vi "getIntersectionFromEnemy-BallLineAndGoalLine.vi"(8 "error in (no error)":errorcluster, 9 "Robot":refnum<class "Robot.lvclass">, 10 "Game":refnum<class "Game.lvclass">, 11 "Utilities in":refnum<class "Utilities.lvclass">) -> (0 "error out":errorcluster, 1 "y_intersection":dbl, 2 "x_intersection":dbl, 3 "Utilities out":refnum<class "Utilities.lvclass">)   [LabVIEW 2018, in "Utilities.lvclass"]
uses:
  Utilities.lvclass
  Robot_class/Robot.lvclass
  C:/Users/Ronaldo/Desktop/Phoenix GIT/SSL_AI/Object_class/Object.lvclass
  Game_class/Game.lvclass
  Game_class/Game.lvclass/Game.ctl
  Object_class/Object.lvclass/Object.ctl
  Game_class/Read FieldRef.vi
  Game_class/Read BallRef.vi
  Object_class/Read x.vi
  Object_class/Read y.vi
  Ball_class/Ball.lvclass
  Field_class/Field.lvclass
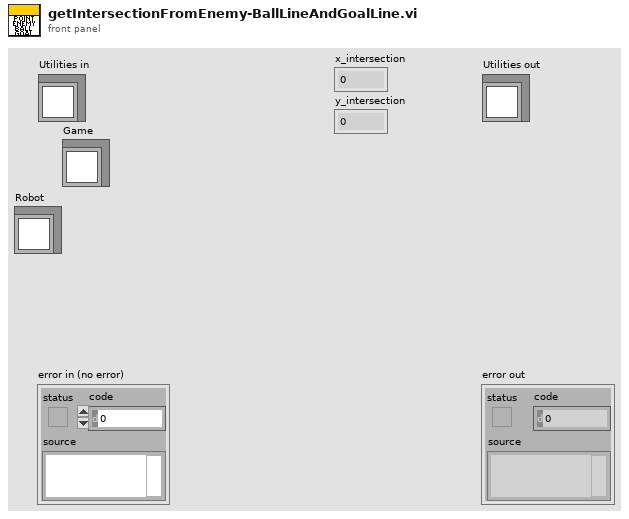
[diagram p1: front panel]
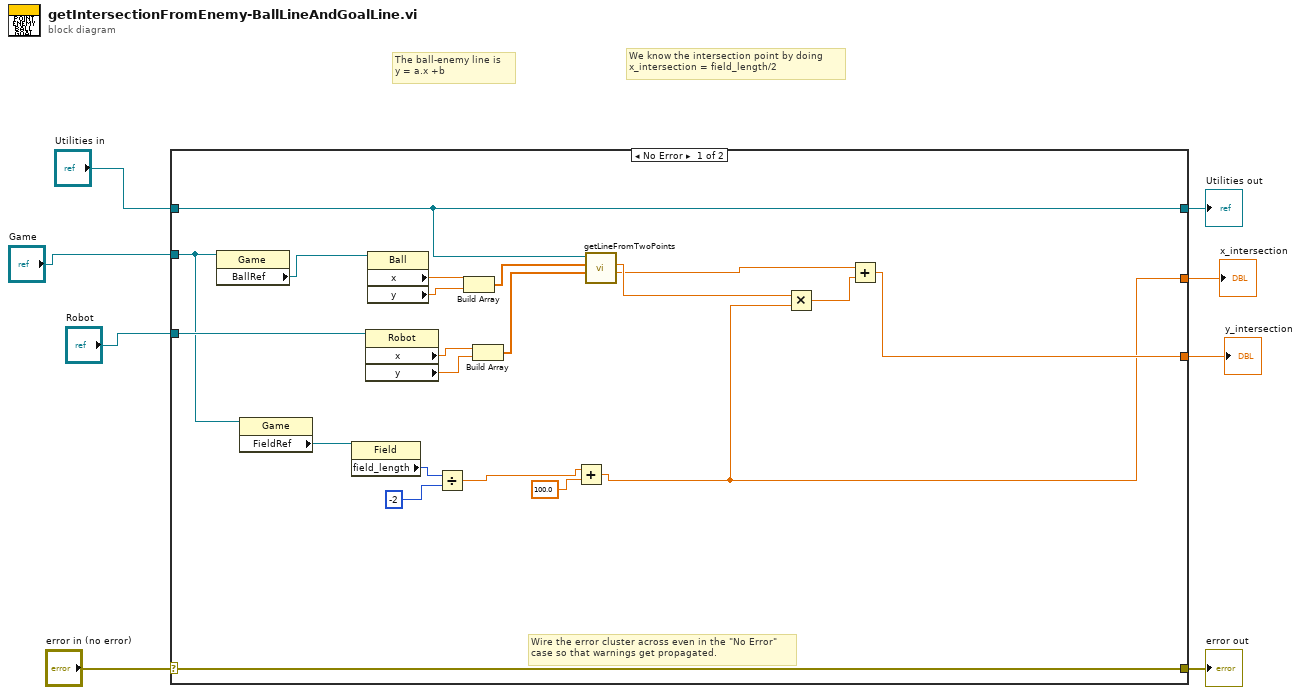
[diagram p0: block diagram]
diagram:
  # "We know the intersection point by doing\nx_intersection = field_length/2"
  # "The ball-enemy line is \ny = a.x +b"
  n1 = case shown="No Error" "error in (no error)" {
    selector: "error in (no error)" -> [w29 w31]
    tunnel: [w29 w31] -> w7
    tunnel: [w21 w30] -> w6
    tunnel: "Utilities in" -> [w21 w30]
    tunnel: "Robot" -> [w22 _]
    tunnel: "Game" -> [w19 _]
    tunnel: [w11 _] -> w2
    tunnel: [w12 _] -> w1
    frame No Error {
      # "Wire the error cluster across even in the \"No Error\"\ncase so that warnings get propagated."
      n2 = property class="Game"(reference=w19) -> ("BallRef"=w20:refnum<class "Ball.lvclass">)  [unwired: 1 in, 2 out]
      n3 = property class="Game"(reference=w19) -> ("FieldRef"=w18:refnum<class "Field.lvclass">)  [unwired: 1 in, 2 out]
      n4 = property class="Field"(reference=w18) -> ("field_length"=w17:i32)  [unwired: 1 in, 2 out]
      n5 = property class="Robot"(reference=w22) -> ("x"=w26:dbl, "y"=w27:dbl)  [unwired: 1 in, 2 out]
      n6 = property class="Ball"(reference=w20) -> ("x"=w23:dbl, "y"=w24:dbl)  [unwired: 1 in, 2 out]
      n7 = Divide(x=w17, y=-2) -> (x/y=w10:dbl)
      n8 = Build Array(w23, w24) -> (w25:dbl[])
      n9 = Build Array(w26, w27) -> (w28:dbl[])
      n10 = Add(x=w10, y=100.0) -> (x+y=w11:dbl)
      n11 = call "getLineFromTwoPoints.vi"("Point 2"=w28, "Point 1"=w25, "Utilities in"=w21) -> ("b"=w13:dbl, "a"=w15:dbl)  [unwired: 5 in, 2 out]
      n12 = Multiply(x=w15, y=w11) -> (x*y=w14:dbl)
      n13 = Add(x=w13, y=w14) -> (x+y=w12:dbl)
    }
    frame Error {
    }
  }
  "error out" <- w7
  "Utilities out" <- w6
  "x_intersection" <- w2
  "y_intersection" <- w1
